vi "Auto_Store_MAIN_rach_final.vi"() -> ()   [LabVIEW 2016]
doc: "自动采集图线程序。\n\n1. 命名只需要给出文件夹目录，base name 可以不写，否则将以 path/base-name1_1.tif，path/base-name1.5_2.tif。后面的 _2 , _1 只有 frames 大于1 才会添加。\n2. start 可以比 end大，自动递减，否则递增。\n3. one pass 表示只以 step 间隔从 start 到 end，选中 auto reverse 可以自动从 end 返回到 start，并在 基名（base name）前 加 bg_。注意 start 减 end 结果除以 step 应是整数。\n4. 每次采集完后需要点击 paused 转到 Continue，继续下一个数据的采集。\n5. force stop 可以强制退出（paused 状态下方可）。\n\n——冉成 2018.09.14"
uses:
  Global.vi
panel:
  in  "Slide":dbl(slide)=0.7000000000000001 min=0.0 max=2.0 step=0.1 scale=0.0..2.0
  out "stop_all":bool
  in  "stop":bool
  in  "w1":i32 min=0 max=2048 step=1
  in  "w2":i32=2048 min=0 max=2048 step=1
  in  "h2":i32=2048 min=0 max=2048 step=1
  in  "h1":i32 min=0 max=2048 step=1
  out "moving":bool
  out "frames_rec":i32
  out "actual":dbl
  in  "Set":dbl=2.0
  in  "Frames":i32=1
  in  "Parameter":u32(ring)=2049184 items=["SENSOR MODE"=4212128, "CCD MODE"=4212384, "READOUT MODE"=4211872, "ACTIVE VIEW INDEX"=4343136, "BITS PER CHANNEL"=4342976, "IMAGE PIXEL TYPE"=4343296, "BINNING"=4215968, "EXPOSURE TIME"=2049184, "CONTRAST GAIN"=3163312, "CONTRAST OFFSET"=3163328, "LIGHT MODE"=2114720, "SENSITIVITY"=2114992, "PHOTON IMAGING MODE"=2115200, "HIGH DYNAMIC RANGE MODE"=3163360, "WHITE BALANCE"=3163568, "TEMPERATURE"=2115232, "TEMPERATURE TARGET"=2115264, "SENSOR COOLER FAN"=2115296, "LINEBUNDLE HEIGHT"=4212192, "MECHANICAL SHUTTER"=2115488, "BACK FOCUS POSITION"=8422304, "TRIGGER CONNECTOR"=1066432, "TRIGGER SOURCE"=1066144, "OUTPUT TRIGGER SOURCE"=1852576, "TRIGGER GLOBAL EXPOSURE"=2049680, "FIRST TRIGGER BEHAVIOR"=2049696, "CHANNEL SYNC"=1852352, "READOUT DIRECTION"=4211904, "PRE HSYNC COUNT"=1852704, "INTERNAL LINE SPEED"=4226000, "INTERNAL LINE INTERVAL"=4226016]
  in  "Clear?":bool
  out "Position":dbl
  in  "反转？":bool
  in  "Mode：":bool=TRUE
  in  "start":bool
  in  "auto convert2tiff":bool=TRUE caption="Blank Button"
  in  "Port":u16=5 caption="芜澳斣崋"
  out "Current_G":i32
  in  "Direction:":bool
  in  "Move steps":i16=1000
  in  "Groups":i32=2 min=0 step=1
  out "DCAM Version":string
  out "cam_status":bool
  out "Lib Version":string
  out "Display":T1(plugin-control)
  in  "Folder Path":path
  # "Default: 5"
  # "1"
  # "2"
  # "仅移动"
  # "测量"
  # "前"
  # "后"
  # "Status"
  # "裁剪图片"
  # "Add delay. units (s)"
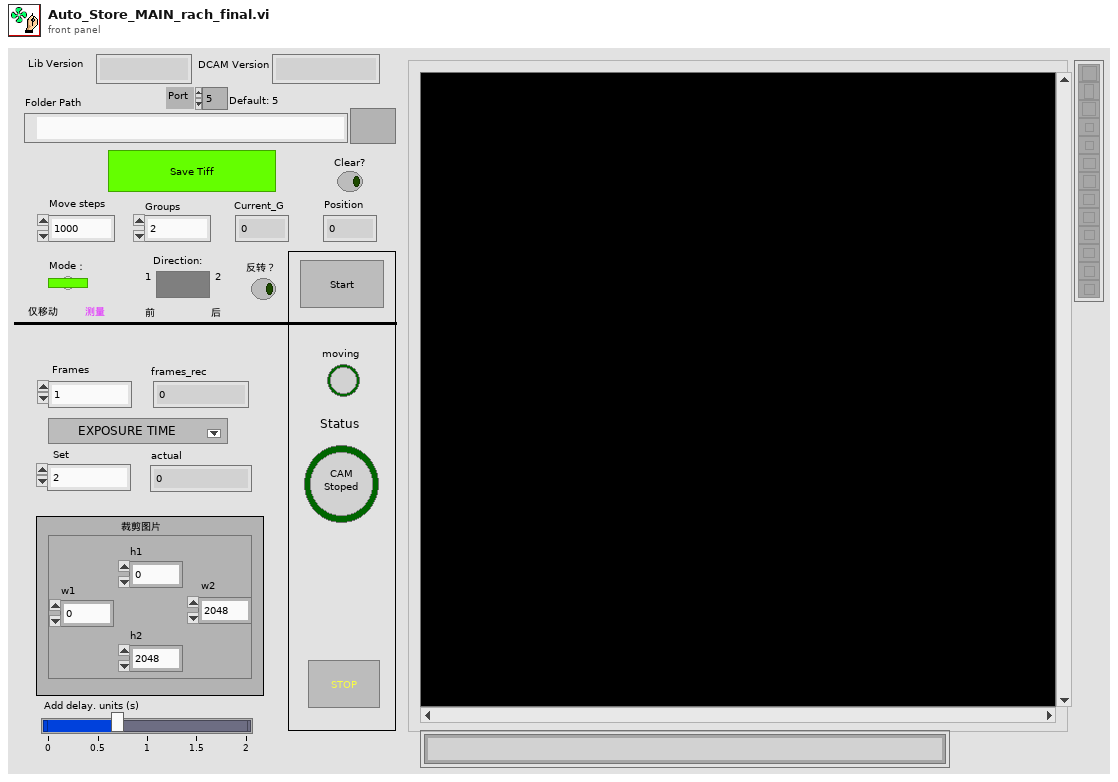
[diagram p1: front panel]
types:
  T1 = typedef "IMAQ Image.ctl" = refnum<image>
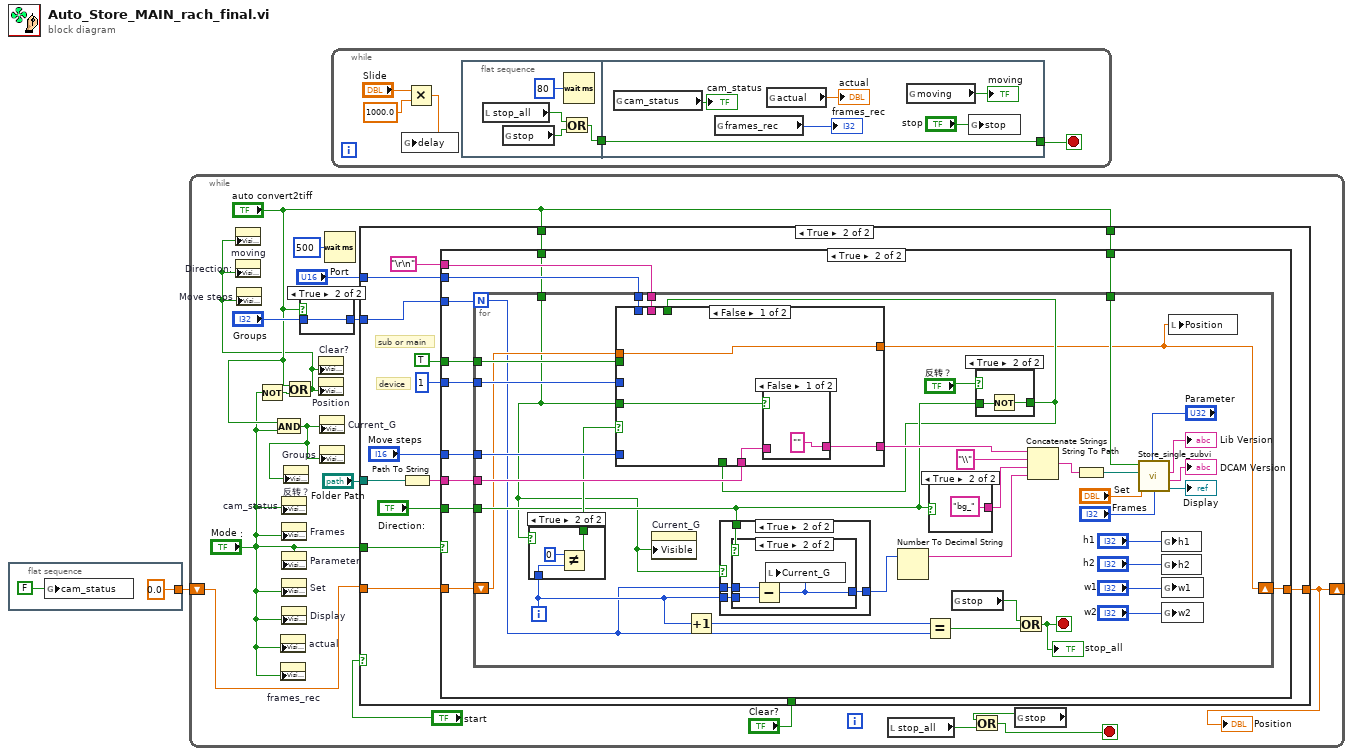
[diagram p0: block diagram]
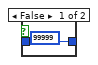
[diagram p2: hidden frame]
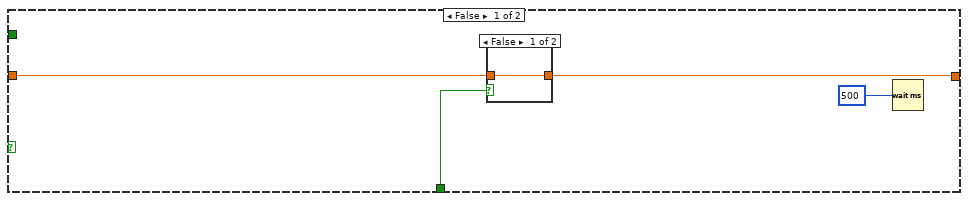
[diagram p3: hidden frame]
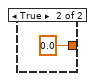
[diagram p4: hidden frame]
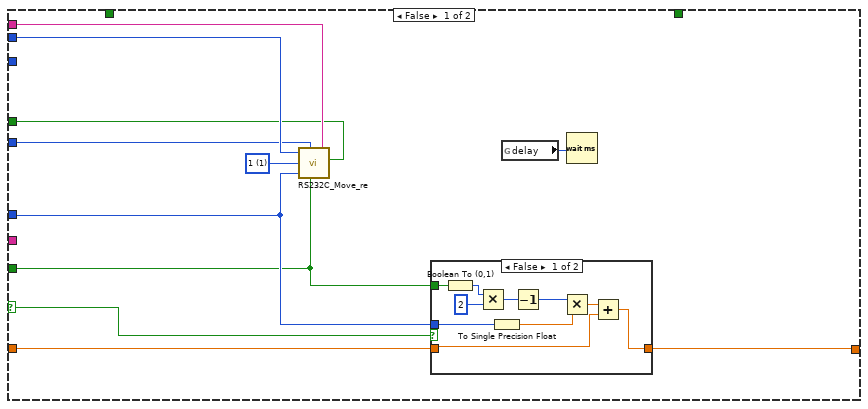
[diagram p5: hidden frame]
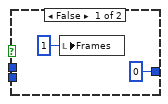
[diagram p7: hidden frame]
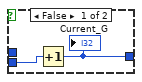
[diagram p8: hidden frame]
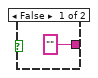
[diagram p10: hidden frame]
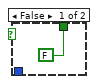
[diagram p11: hidden frame]
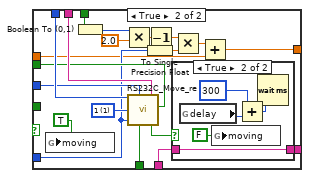
[diagram p13: hidden frame]
diagram:
  n1 = flat-sequence {
    tunnel: [0.0] -> w1
    frame #0 {
      n2 = global write "Global.vi" "cam_status"(FALSE) -> ()
    }
  }
  n3 = while {
    shift-right: [w16] -> _
    shift-left: w1 -> [w17]
    stop <- w4 stop-if-true
    n4 = Not(x="Mode：") -> (.not. x?=w9:bool)
    n5 = And(x="auto convert2tiff", y="Mode：") -> (x .and. y?=w6:bool)
    n6 = property on="actual" class="DigNum (strict)"("Visible"="Mode：") -> ()  [unwired: 2 in, 2 out]
    n7 = property on="frames_rec" class="DigNum (strict)"("Visible"="Mode：") -> ()  [unwired: 2 in, 2 out]
    n8 = property on="cam_status" class="Bool (strict)"("Visible"="Mode：") -> ()  [unwired: 2 in, 2 out]
    n9 = property on="Frames" class="DigNum (strict)"("Visible"="Mode：") -> ()  [unwired: 2 in, 2 out]
    n10 = property on="Parameter" class="Ring (strict)"("Visible"="Mode：") -> ()  [unwired: 2 in, 2 out]
    n11 = property on="Set" class="DigNum (strict)"("Visible"="Mode：") -> ()  [unwired: 2 in, 2 out]
    n12 = property on="Display" class="ImageControl"("Visible"="Mode：") -> ()  [unwired: 2 in, 2 out]
    n13 = property on="反转？" class="Bool (strict)"("Visible"=w6) -> ()  [unwired: 2 in, 2 out]
    n14 = Or(x="auto convert2tiff", y=w9) -> (x .or. y?=w5:bool)
    n15 = property on="moving" class="Bool (strict)"("Visible"=w5) -> ()  [unwired: 2 in, 2 out]
    n16 = property on="Direction:" class="Bool (strict)"("Visible"=w5) -> ()  [unwired: 2 in, 2 out]
    n17 = property on="Move steps" class="DigNum (strict)"("Visible"=w5) -> ()  [unwired: 2 in, 2 out]
    n18 = case shown="True" "auto convert2tiff" {
      tunnel: [99999 ("Groups") w22] -> w14
      tunnel: "Groups" -> [_ w22]
      frame False {
      }
      frame True {
      }
    }
    n19 = property on="Clear?" class="Bool"("Visible"=w5) -> ()  [unwired: 2 in, 2 out]
    n20 = property on="Position" class="DigNum (strict)"("Visible"=w5) -> ()  [unwired: 2 in, 2 out]
    n21 = property on="Current_G" class="DigNum (strict)"("Visible"=w6) -> ()  [unwired: 2 in, 2 out]
    n22 = property on="Groups" class="DigNum (strict)"("Visible"=w6) -> ()  [unwired: 2 in, 2 out]
    n23 = Wait (ms)(milliseconds to wait=u32 500) -> ()  [unwired: 1 out]
    n24 = case shown="True" "start" {
      tunnel: "Folder Path" -> [_ w39]
      tunnel: w14 -> [_ w42]
      tunnel: "Mode：" -> [_ w33]
      tunnel: "Port" -> [_ w30]
      tunnel: w17 -> [w24 w35]
      tunnel: [w23 w34] -> w16
      tunnel: "Clear?" -> [w25 _]
      tunnel: "auto convert2tiff" -> [_ w32]
      tunnel: "auto convert2tiff" -> [_ w31]
      frame False {
        n25 = case shown="False" w25 {
          tunnel: w24 -> [w27 _]
          tunnel: [w27 0.0] -> w23
          frame False {
          }
          frame True {
          }
        }
        n26 = Wait (ms)(milliseconds to wait=u32 500) -> ()  [unwired: 1 out]
      }
      frame True {
        # "device"
        # "sub or main"
        n27 = Path To String(path=w39) -> (string=w38:string)
        n28 = case shown="True" w33 {
          selector: w33 -> [w46 _]
          tunnel: w38 -> [_ w76]
          tunnel: "Direction:" -> [w47 w75]
          tunnel: "Move steps" -> [w48 w74]
          tunnel: w42 -> [_ w73]
          tunnel: w30 -> [w52 w72]
          tunnel: "\r\n" -> [w51 w71]
          tunnel: 1 -> [w49 w70]
          tunnel: TRUE -> [w50 w69]
          tunnel: w35 -> [w45 w68]
          tunnel: [w44 w67] -> w34
          tunnel: w32 -> [_ w66]
          tunnel: w31 -> [_ w65]
          frame False {
            w53 = u8 1 items=["0", "1", "2", "3", "4"] ("Axis Number")
            n29 = call "RS232C_Move_re.vi"("Port Number"=w52, "Axis Count"=w49, "Axis Number"=w53, "Pulse Number"=w48, "Direction"=w47, "Delimiter"=w51, "Main/Sub"=w50) -> ()  [unwired: 2 out]
            n30 = case shown="False" w46 {
              tunnel: w48 -> [w60 _]
              tunnel: w47 -> [w59 _]
              tunnel: [w54 w64] -> w44
              tunnel: w45 -> [w55 w64]
              frame False {
                n31 = Boolean To (0,1)(Boolean=w59) -> (0, 1=w63:i16)
                n32 = Multiply(x=w63, y=2) -> (x*y=w61:i32)
                n33 = To Single Precision Float(number=w60) -> (single precision float=w57:sgl)
                n34 = Decrement(x=w61) -> (x-1=w58:i32)
                n35 = Multiply(x=w58, y=w57) -> (x*y=w56:sgl)
                n36 = Add(x=w56, y=w55) -> (x+y=w54:dbl)
              }
              frame True {
              }
            }
            n37 = global read "Global.vi" "delay"() -> (w43:i32)
            n38 = Wait (ms)(milliseconds to wait=w43) -> ()  [unwired: 1 out]
          }
          frame True {
            n39 = for {
              N: w73 -> [w88]
              tunnel: w76 -> [w112]
              tunnel: w66 -> [w108]
              tunnel: w74 -> [w113]
              tunnel: w75 -> [w96]
              tunnel: w65 -> [w80]
              tunnel: w72 -> [w95]
              tunnel: w71 -> [w94]
              tunnel: w70 -> [w93]
              tunnel: w69 -> [w92]
              shift-right: [w86] -> w67
              shift-left: w68 -> [w91]
              i -> [w89]
              stop <- w78 stop-if-true
              n40 = case shown="True" w80 {
                tunnel: w89 -> [_ w132]
                tunnel: [FALSE w131] -> w107
                frame False {
                }
                frame True {
                  n41 = Not Equal?(x=0 ("y"), y=w132) -> (x != y?=w131:bool)
                }
              }
              n42 = property on="Current_G" class="DigNum (strict)"("Visible"=w80) -> ()  [unwired: 2 in, 2 out]
              n43 = Increment(x=w89) -> (x+1=w106:i32)
              n44 = case shown="True" w80 {
                tunnel: [0 w119] -> w109
                tunnel: w89 -> [_ w118]
                tunnel: w96 -> [_ w117]
                tunnel: w88 -> [_ w116]
                frame False {
                  n45 = local write "Frames"(1 ("Frames")) -> ()
                }
                frame True {
                  n46 = case shown="True" w117 {
                    tunnel: w118 -> [w121 w124]
                    tunnel: [w120 w122] -> w119
                    tunnel: w116 -> [_ w123]
                    frame False {
                      n47 = Increment(x=w121) -> (x+1=w120:i32)
                      "Current_G" <- w120
                    }
                    frame True {
                      n48 = Subtract(x=w123, y=w124) -> (x-y=w122:i32)
                      n49 = local write "Current_G"(w122) -> ()
                    }
                  }
                }
              }
              n50 = Number To Decimal String(number=w109) -> (decimal integer string=w110:string)  [unwired: 1 in]
              n51 = Equal?(x=w106, y=w88) -> (x = y?=w79:bool)
              n52 = case shown="True" w96 {
                tunnel: ["" ("string") "bg_" ("string")] -> w98
                frame False {
                }
                frame True {
                }
              }
              n53 = global read "Global.vi" "stop"() -> (w77:bool)
              n54 = case shown="True" "反转？" {
                tunnel: w96 -> [w125 w127]
                tunnel: [w125 w126] -> w90
                frame False {
                }
                frame True {
                  n55 = Not(x=w127) -> (.not. x?=w126:bool)
                }
              }
              n56 = case shown="False" w107 {
                tunnel: w113 -> [_ w146]
                tunnel: w112 -> [w135 w157]
                tunnel: [w137 w156] -> w111
                tunnel: w90 -> [_ w144]
                tunnel: w80 -> [w136 _]
                tunnel: w95 -> [_ w155]
                tunnel: w94 -> [_ w154]
                tunnel: w93 -> [_ w153]
                tunnel: w92 -> [_ w152]
                tunnel: [w134 w145] -> w86
                tunnel: w91 -> [w134 w141]
                tunnel: w90 -> [_ w143]
                frame False {
                  n57 = case shown="False" w136 {
                    tunnel: ["" w139] -> w137
                    tunnel: w135 -> [_ w139]
                    frame False {
                    }
                    frame True {
                    }
                  }
                }
                frame True {
                  w159 = u8 1 items=["0", "1", "2", "3", "4"] ("Axis Number")
                  n58 = global write "Global.vi" "moving"(TRUE ("Moved？")) -> ()
                  n59 = Boolean To (0,1)(Boolean=w143) -> (0, 1=w147:i16)
                  n60 = Multiply(x=w147, y=2.0) -> (x*y=w149:dbl)
                  n61 = call "RS232C_Move_re.vi"("Port Number"=w155, "Axis Count"=w153, "Axis Number"=w159, "Pulse Number"=w146, "Direction"=w144, "Delimiter"=w154, "Main/Sub"=w152) -> ("OK Done"=w158:bool)  [unwired: 1 out]
                  n62 = To Single Precision Float(number=w146) -> (single precision float=w151:sgl)
                  n63 = Decrement(x=w149) -> (x-1=w150:dbl)
                  n64 = case shown="True" w158 {
                    tunnel: w157 -> [w160 w165]
                    tunnel: [w160 w165] -> w156
                    frame False {
                    }
                    frame True {
                      n65 = global read "Global.vi" "delay"() -> (w161:i32)
                      n66 = global write "Global.vi" "moving"(FALSE ("Moving？")) -> ()
                      n67 = Add(x=u32 300 ("milliseconds to wait"), y=w161) -> (x+y=w163:u32)
                      n68 = Wait (ms)(milliseconds to wait=w163) -> ()  [unwired: 1 out]
                    }
                  }
                  n69 = Multiply(x=w150, y=w151) -> (x*y=w142:dbl)
                  n70 = Add(x=w142, y=w141) -> (x+y=w145:dbl)
                }
              }
              n71 = Or(x=w77, y=w79) -> (x .or. y?=w78:bool)
              "stop_all" <- w78
              n72 = Concatenate Strings(w111, "\\" ("string"), w98, w110) -> (w103:string)
              n73 = String To Path(string=w103) -> (path=w104:path)
              n74 = call "Store_single_subvi.vi"("Parameter"="Parameter", "Set"="Set", "Frames"="Frames", "File"=w104, "save"=w108) -> ("Display"=→"Display":T1, "DCAM Version"=→"DCAM Version":string, "Library Version"=→"Lib Version":string)
              n75 = global write "Global.vi" "h1"("h1") -> ()
              n76 = global write "Global.vi" "h2"("h2") -> ()
              n77 = global write "Global.vi" "w1"("w1") -> ()
              n78 = global write "Global.vi" "w2"("w2") -> ()
              n79 = local write "Position"(w86) -> ()
            }
          }
        }
      }
    }
    "Position" <- w16
    n80 = local read "stop_all"() -> (w11:bool)
    n81 = global read "Global.vi" "stop"() -> (w10:bool)
    n82 = Or(x=w10, y=w11) -> (x .or. y?=w4:bool)
  }
  n83 = while {
    stop <- w166 stop-if-true
    n84 = Multiply(x="Slide", y=1000.0) -> (x*y=w167:dbl)
    n85 = global write "Global.vi" "delay"(w167) -> ()
    n86 = flat-sequence {
      tunnel: [w172] -> w170
      tunnel: w170 -> [w177]
      tunnel: [w177] -> w166
      frame #0 {
        n87 = local read "stop_all"() -> (w171:bool)
        n88 = global read "Global.vi" "stop"() -> (w173:bool)
        n89 = Or(x=w171, y=w173) -> (x .or. y?=w172:bool)
        n90 = Wait (ms)(milliseconds to wait=u32 80) -> ()  [unwired: 1 out]
      }
      frame #1 {
        n91 = global read "Global.vi" "cam_status"() -> (→"cam_status":bool)
        n92 = global read "Global.vi" "frames_rec"() -> (→"frames_rec":i32)
        n93 = global read "Global.vi" "actual"() -> (→"actual":dbl)
        n94 = global read "Global.vi" "moving"() -> (→"moving":bool)
        n95 = global write "Global.vi" "stop"("stop") -> ()
      }
    }
  }
